vi "Create_Heater_Setpoints_File.vi"(4 "Mode":enum16{"Load from File", "Save to File"}(ring), 8 "Filename":path) -> ()   [LabVIEW 2011]
uses:
  ADAM Client/Sub VIs/Heater_Setpoint.ctl
  ADAM Client/Sub VIs/ADAM Controls/Channel_names.ctl
panel:
  out "Setpoints Out":T1[](array[typedef])
  in  "Setpoints In":T1[](array[typedef])
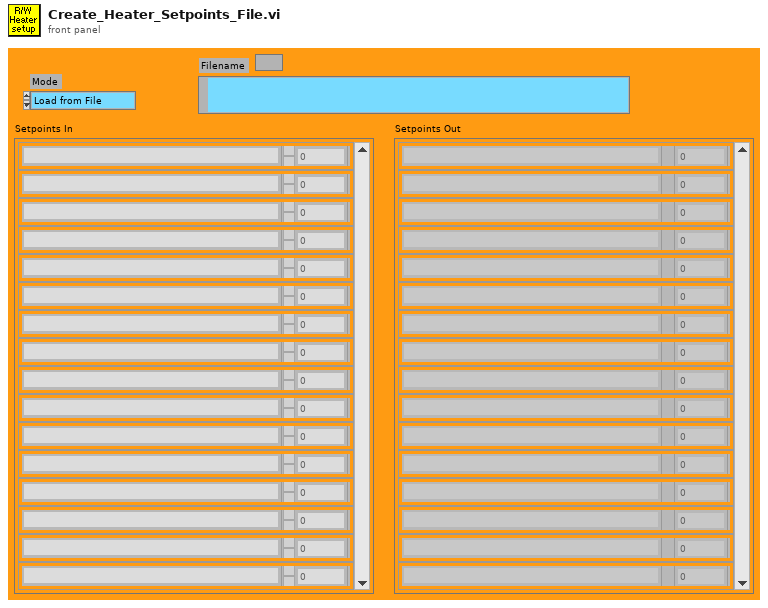
[diagram p1: front panel]
types:
  T1 = typedef "Heater_Setpoint.ctl" = cluster{"Ch Name":string, "Setpoint":dbl}
  T2 = typedef "Channel_names.ctl" = enum16{"Active Only", "Active + Off", "All Channels"}
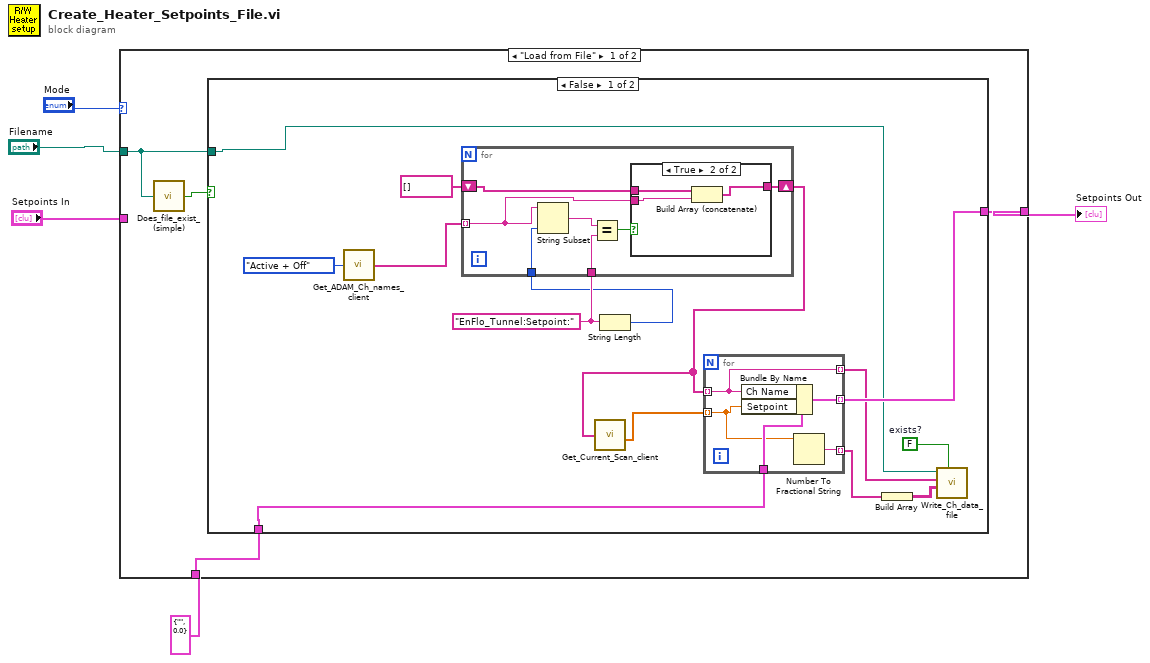
[diagram p0: block diagram]
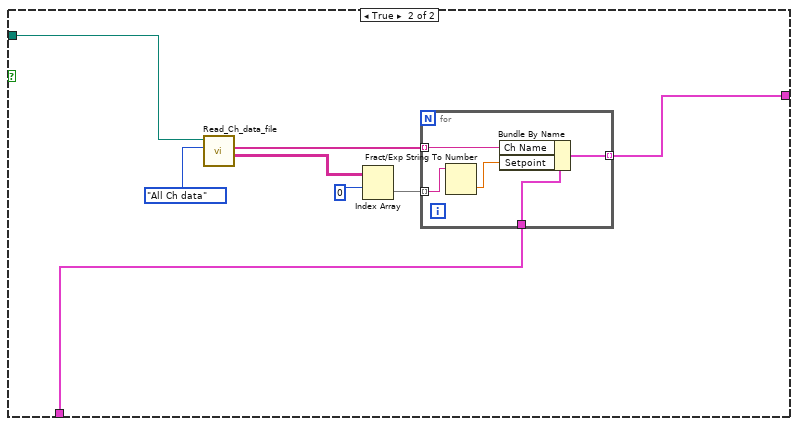
[diagram p3: hidden frame]
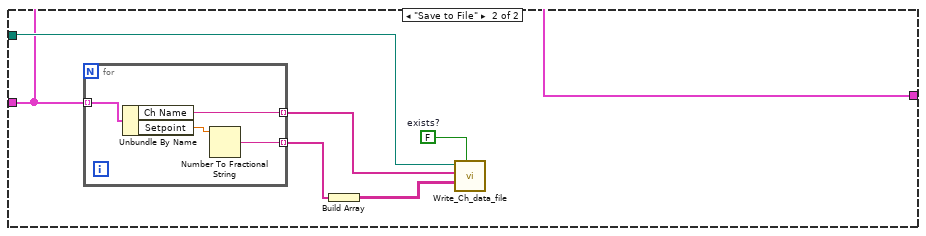
[diagram p4: hidden frame]
diagram:
  n1 = case shown="\"Load from File\"" "Mode" {
    tunnel: "Filename" -> [w7 w58]
    tunnel: T1 {"Ch Name"="", "Setpoint"=0.0} ("Cluster") -> [w9 _]
    tunnel: [w8 w53] -> w2
    tunnel: "Setpoints In" -> [_ w53]
    frame "Load from File" {
      n2 = call "Does_file_exist_(simple).vi"("Pathname"=w7) -> ("exists?"=w6:bool)
      n3 = case shown="False" w6 {
        tunnel: w9 -> [w15 w47]
        tunnel: [w18 w46] -> w8
        tunnel: w7 -> [w10 w45]
        frame False {
          w13 = FALSE  # exists?
          w21 = "EnFlo_Tunnel:Setpoint:"
          n4 = call "Get_ADAM_Ch_names_client.vi"("Channel names set"=Channel_names."Active + Off") -> ("Ch names"=w19:string[])
          n5 = String Length(string=w21) -> (length=w20:i32)
          n6 = for {
            shift-right: [w29] -> w17
            shift-left: string[] [] -> [w31]
            tunnel: w19 -> [w30] mode=indexing
            tunnel: w20 -> [w35]
            tunnel: w21 -> [w34]
            n7 = String Subset(string=w30, length (rest)=w35) -> (substring=w33:string)  [unwired: 1 out]
            n8 = Equal?(x=w33, y=w34) -> (x = y?=w32:bool)
            n9 = case shown="True" w32 {
              tunnel: w31 -> [w36 w39]
              tunnel: w30 -> [_ w38]
              tunnel: [w36 w37] -> w29
              frame False {
              }
              frame True {
                n10 = Build Array (concatenate)(w39, w38) -> (w37:string[])
              }
            }
          }
          n11 = call "Get_Current_Scan_client.vi"("ADAM Ch Names"=w17) -> ("Numerical Values"=w16:dbl[])  [unwired: 1 in, 2 out]
          n12 = for {
            tunnel: w15 -> [w28]
            tunnel: w17 -> [w25] mode=indexing
            tunnel: [w27] -> w18 mode=indexing
            tunnel: w16 -> [w26] mode=indexing
            tunnel: [w25] -> w12 mode=indexing
            tunnel: [w24] -> w11 mode=indexing
            n13 = Bundle By Name(cluster=w28, "Ch Name"=w25, "Setpoint"=w26) -> (w27:T1)
            n14 = Number To Fractional String(number=w26) -> (F-format string=w24:string)  [unwired: 3 out]
          }
          n15 = Build Array(w11) -> (w14:string[][])
          n16 = call "Write_Ch_data_file.vi"("exists?"=w13, "Channel Values"=w14, "Channel names"=w12, "Filename"=w10) -> ()  [unwired: 4 in, 4 out]
        }
        frame True {
          n17 = call "Read_Ch_data_file.vi"("Output"=enum16{"All Ch data", "The last few rows"}."All Ch data", "Filename"=w45) -> ("Channel Values"=w40:string[][], "Merged Channels"=w41:string[])  [unwired: 3 in, 3 out]
          n18 = Index Array(array=w40, index (row)=0 ("Index")) -> (element=w43:string[])  [unwired: 1 in]
          n19 = for {
            tunnel: w47 -> [w52]
            tunnel: w41 -> [w51] mode=indexing
            tunnel: w43 -> [w50] mode=indexing
            tunnel: [w48] -> w46 mode=indexing
            n20 = Fract/Exp String To Number(string=w50) -> (number=w49:dbl)  [unwired: 4 out]
            n21 = Bundle By Name(cluster=w52, "Ch Name"=w51, "Setpoint"=w49) -> (w48:T1)
          }
        }
      }
    }
    frame "Save to File" {
      w57 = FALSE  # exists?
      n22 = for {
        tunnel: w53 -> [w62] mode=indexing
        tunnel: [w60] -> w55 mode=indexing
        tunnel: [w59] -> w54 mode=indexing
        n23 = Unbundle By Name(w62) -> ("Ch Name"=w59:string, "Setpoint"=w61:dbl)
        n24 = Number To Fractional String(number=w61) -> (F-format string=w60:string)  [unwired: 3 out]
      }
      n25 = Build Array(w55) -> (w56:string[][])
      n26 = call "Write_Ch_data_file.vi"("exists?"=w57, "Channel Values"=w56, "Channel names"=w54, "Filename"=w58) -> ()  [unwired: 4 in, 4 out]
    }
  }
  "Setpoints Out" <- w2
